vi "If AND Then Else.vi"(7 "AND 조건":bool, 8 "AND 조건 텍스트":string, 9 "현재 텍스트":string) -> (3 "현재 텍스트 출력":string)   [LabVIEW 2010]
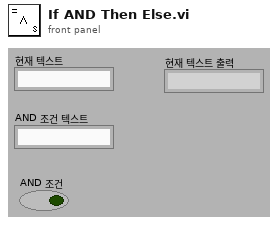
[diagram p1: front panel]
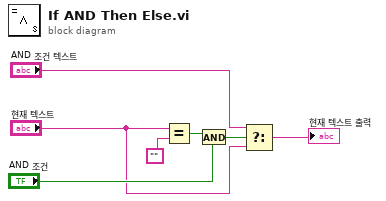
[diagram p0: block diagram]
diagram:
  n1 = Equal?(x="현재 텍스트", y="") -> (x = y?=w3:bool)
  n2 = And(x=w3, y="AND 조건") -> (x .and. y?=w5:bool)
  n3 = Select(t="AND 조건 텍스트", s=w5, f="현재 텍스트") -> (s? t:f=→"현재 텍스트 출력":string)
